vi "stopService.vi"(8 "error in (no error)":errorcluster, 11 "Communicator in":refnum<class "Communicator.lvclass">) -> (0 "error out":errorcluster, 3 "Communicator out":refnum<class "Communicator.lvclass">)   [LabVIEW 2016, in "M1M3SupportCommunicator.lvlib" / "Communicator.lvclass"]
uses:
  Communicator.lvclass
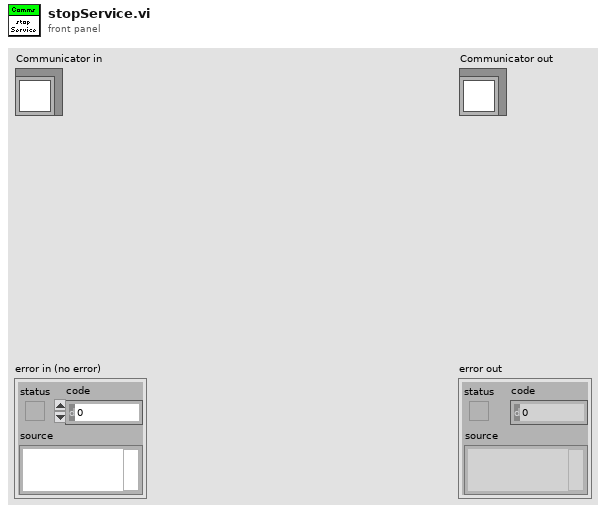
[diagram p1: front panel]
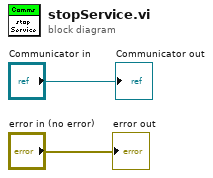
[diagram p0: block diagram]
diagram:
  "error out" <- "error in (no error)"
  "Communicator out" <- "Communicator in"
